vi "Get Session from ClientID.vi"(8 "error in (no error)":errorcluster, 10 "Client ID":string, 11 "Server in":refnum<class "Server.lvclass">) -> (0 "error out":errorcluster, 1 "found?":bool, 2 "SessionMailbox":refnum<queue>, 3 "Server out":refnum<class "Server.lvclass">)   [LabVIEW 2013, in "MQTT Server.lvlib" / "Server.lvclass"]
uses:
  Server.lvclass
  Response -- cluster.ctl
  Control Packets/ControlPacket/ControlPacket.lvclass
  Server.lvclass/Server.ctl
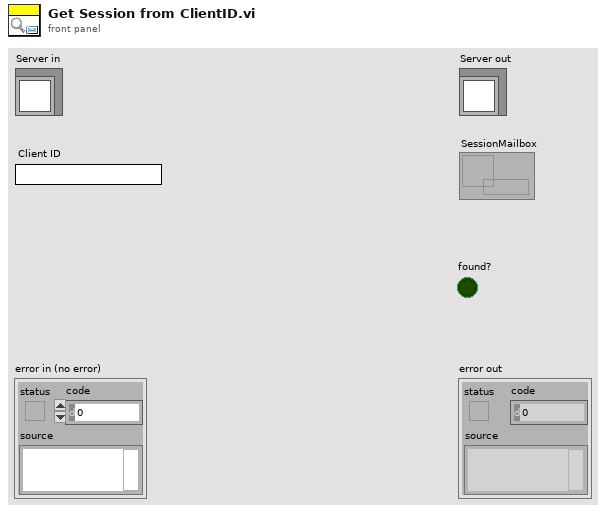
[diagram p1: front panel]
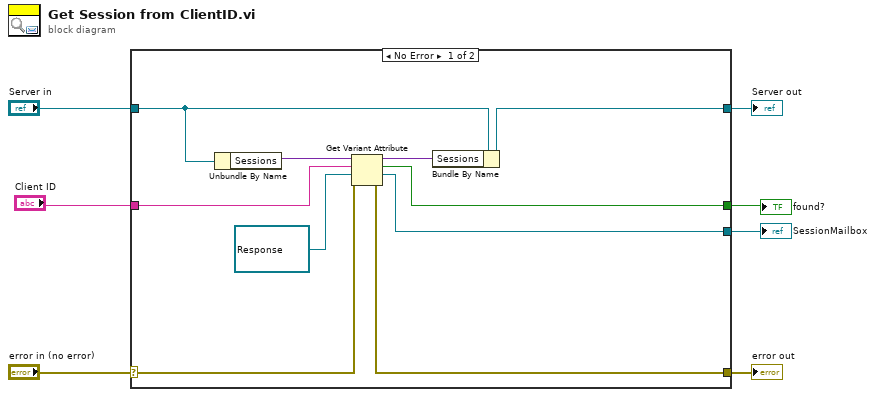
[diagram p0: block diagram]
diagram:
  n1 = case shown="No Error" "error in (no error)" {
    selector: "error in (no error)" -> [w15 w19]
    tunnel: [w14 w19] -> w6
    tunnel: [w11 w18] -> w4
    tunnel: "Server in" -> [w12 w18]
    tunnel: "Client ID" -> [w16 _]
    tunnel: [w10 _] -> w2
    tunnel: [w8 _] -> w1
    frame No Error {
      n2 = Unbundle By Name(w12) -> ("Sessions"=w17:variant)
      n3 = Get Variant Attribute(Variant=w17, name=w16, default value (empty Variant)=refnum<queue> refnum ("SessionMailbox"), error in=w15) -> (duplicate Variant=w13:variant, found=w10:bool, value=w8:refnum<queue>, error out=w14:errorcluster)
      n4 = Bundle By Name(cluster=w12, "Sessions"=w13) -> (w11:refnum<class "Server.lvclass">)
    }
    frame Error {
    }
  }
  "error out" <- w6
  "Server out" <- w4
  "SessionMailbox" <- w1
  "found?" <- w2
